vi "where are we (accelrator, gyro).vi"(9 "Rotation":dbl(knob) scale=0.0..360.0, 10 "Acceleration Y":dbl(slide) scale=-2.0..2.0, 11 "Acceleration X":dbl(slide) scale=-2.0..2.0) -> (3 "appended array":cluster{"[0]":dbl, "[1]":dbl}[](array[cluster]))   [LabVIEW 2014]
panel:
  in  "stop":bool
  out "Position Y":dbl
  out "Position X":dbl
  in  "Wait Time":dbl
  out "XY Graph":cluster{"X":dbl, "Y":dbl}[](graph)
  out "Velocity Y":dbl
  out "Velocity X":dbl
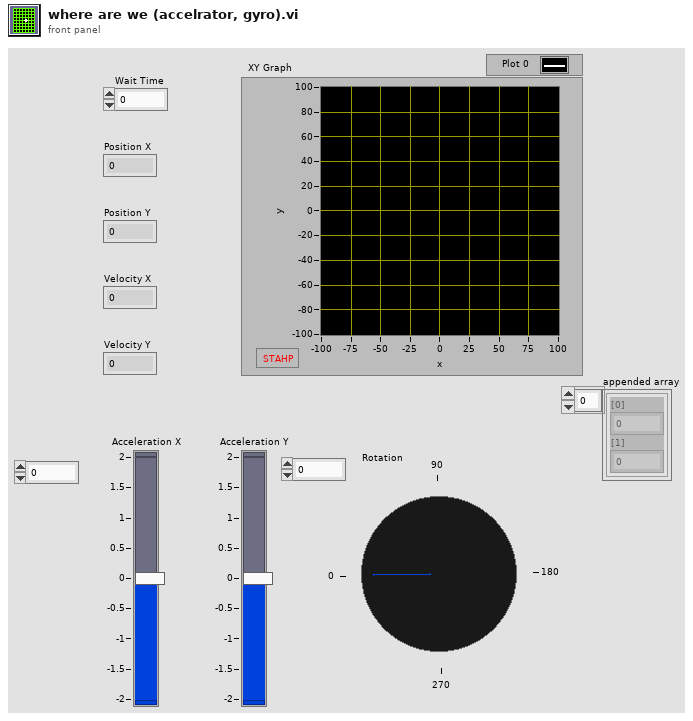
[diagram p1: front panel]
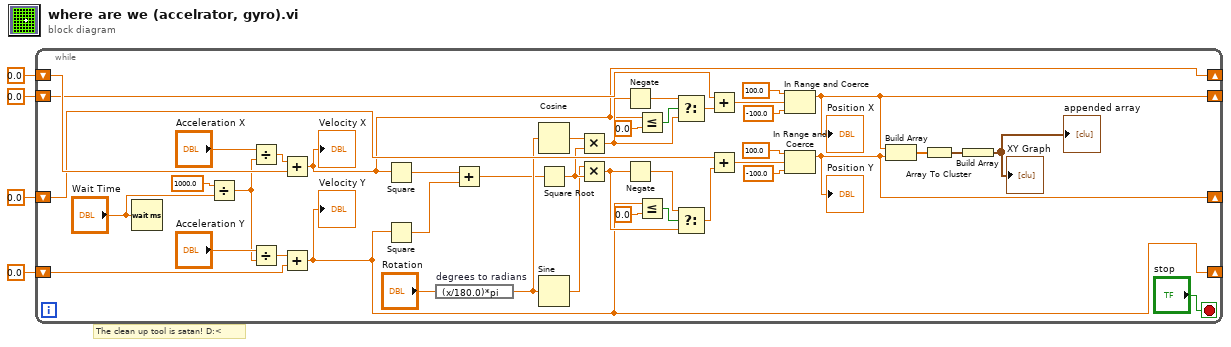
[diagram p0: block diagram]
diagram:
  # "The clean up tool is satan! D:<"
  n1 = while {
    shift-right: [w6] -> _
    shift-left: 0.0 -> [w45]
    shift-right: [w5] -> _
    shift-left: 0.0 -> [w40]
    shift-right: [w31] -> _
    shift-left: 0.0 ("upper limit") -> [w35]
    shift-right: [w27] -> _
    shift-left: 0.0 ("upper limit") -> [w36]
    stop <- "stop" stop-if-true
    n2 = Wait (ms)(milliseconds to wait="Wait Time") -> ()  [unwired: 1 out]
    n3 = Divide(x=1000.0, y="Wait Time") -> (x/y=w42:dbl)
    n4 = Divide(x="Acceleration X", y=w42) -> (x/y=w46:dbl)
    n5 = Divide(x="Acceleration Y", y=w42) -> (x/y=w41:dbl)
    n6 = Add(x=w46, y=w45) -> (x+y=w6:dbl)
    "Velocity X" <- w6
    n7 = Add(x=w41, y=w40) -> (x+y=w5:dbl)
    "Velocity Y" <- w5
    n8 = Square(x=w6) -> (x^2=w22:dbl)
    n9 = Square(x=w5) -> (x^2=w21:dbl)
    n10 = expression code="(x/180.0)*pi" "degrees to radians"("Rotation") -> (w25:dbl)
    n11 = Add(x=w22, y=w21) -> (x+y=w23:dbl)
    n12 = Cosine(x=w25) -> (cos(x)=w20:dbl)
    n13 = Square Root(x=w23) -> (sqrt(x)=w19:dbl)
    n14 = Sine(x=w25) -> (sin(x)=w18:dbl)
    n15 = Multiply(x=w20, y=w19) -> (x*y=w8:dbl)
    n16 = Multiply(x=w18, y=w19) -> (x*y=w14:dbl)
    n17 = Negate(x=w8) -> (-x=w12:dbl)
    n18 = Negate(x=w14) -> (-x=w15:dbl)
    n19 = Less Or Equal?(x=w6, y=0.0) -> (x <= y?=w10:bool)
    n20 = Less Or Equal?(x=w5, y=0.0) -> (x <= y?=w16:bool)
    n21 = Select(t=w12, s=w10, f=w8) -> (s? t:f=w9:dbl)
    n22 = Select(t=w15, s=w16, f=w14) -> (s? t:f=w13:dbl)
    n23 = Add(x=w36, y=w9) -> (x+y=w28:dbl)
    n24 = Add(x=w35, y=w13) -> (x+y=w32:dbl)
    n25 = In Range and Coerce(upper limit=100.0, x=w28, lower limit=-100.0) -> (coerced(x)=w27:dbl)  [unwired: 1 out]
    "Position X" <- w27
    n26 = In Range and Coerce(upper limit=100.0, x=w32, lower limit=-100.0) -> (coerced(x)=w31:dbl)  [unwired: 1 out]
    "Position Y" <- w31
    n27 = Build Array(w27, w31) -> (w39:dbl[])
    n28 = Array To Cluster(array=w39) -> (cluster=w38:cluster{"[0]":dbl, "[1]":dbl})
    n29 = Build Array(w38) -> (→"XY Graph" →"appended array":cluster{"[0]":dbl, "[1]":dbl}[])
  }
